vi "PH_Names.File Extention Setter.vi"(3 "error in (no error)":errorcluster, 4 "File Type":T1="*.tif", 5 "start path (O:\\)":path=path "O:/") -> (0 "error out":errorcluster, 1 "path with extension":path, 2 "cancelled?":bool)   [LabVIEW 2014, in "PH_Common.lvlib"]
doc: "This VI sets a file path with extention to the name chosen."
uses:
  PH_Common.lvlib
  PH_Names.File Types.ctl
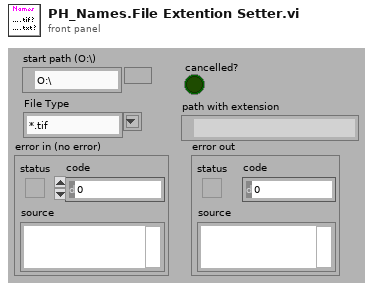
[diagram p1: front panel]
types:
  T1 = typedef "PH_Common.lvlib/PH_Names.File Types.ctl" = string
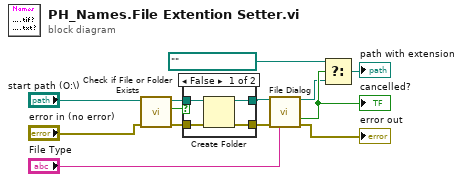
[diagram p0: block diagram]
diagram:
  n1 = call <vilib>:"Check if File or Folder Exists.vi"("error in (no error)"="error in (no error)", "path"="start path (O:\\)") -> ("error out"=w13:errorcluster, "file or folder exists?"=w9:bool, "dup path"=w11:path)  [unwired: 7 in]
  n2 = case shown="False" w9 {
    tunnel: w13 -> [w16 w18]
    tunnel: w11 -> [w17 w19]
    tunnel: [w14 w19] -> w10
    tunnel: [w15 w18] -> w12
    frame False {
      n3 = Create Folder(path (use dialog)=w17, error in=w16) -> (created path=w14:path, error out=w15:errorcluster)  [unwired: 1 in, 1 out]
    }
    frame True {
    }
  }
  n4 = call "File Dialog"("start path"=w10, "error in"=w12, "pattern (all files)"="File Type") -> ("selected path"=w3:path, "cancelled"=w4:bool, "error out"=→"error out":errorcluster)  [unwired: 9 in, 1 out]
  "cancelled?" <- w4
  n5 = Select(t=path "" ("selected path 2"), s=w4, f=w3) -> (s? t:f=→"path with extension":path)
